vi "InTake Set.vi"(1 "InTake Global Data In":T1) -> (0 "InTake Global Data Out":T1)   [LabVIEW 2013]
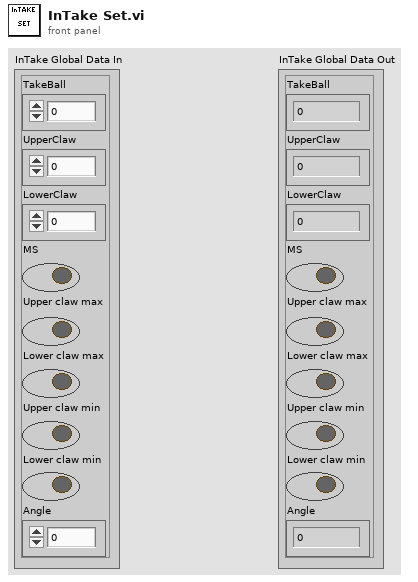
[diagram p1: front panel]
types:
  T1 = cluster{"TakeBall":dbl, "UpperClaw":dbl, "LowerClaw":dbl, "MS":bool, "Upper claw max":bool, "Lower claw max":bool, "Upper claw min":bool, "Lower claw min":bool, "Angle":dbl}
  T2 = typedef "WPI_MotorControlDeviceRef.ctl" = cluster{"DeviceStatus":errorcluster, "Type":enum16{"PWM", "CAN"}, "PWM":cluster{"Digital Module":T3, "PWM Channel":T4, "DeadBand":T5}, "CAN":cluster{"Device Number":u8, "Control Mode":T6, "Semaphore":T7, "Max Vout":dbl}, "Invert":bool, "TransformRef":T8, "InvTransformRef":T8}
  T3 = typedef "FPGA_TypedefDigitalModule.ctl" = enum16{"Digital Module 1", "Digital Module 2"}
  T4 = typedef "FPGA_DIOPWMChannel.ctl" = enum8{"PWM 1", "PWM 2", "PWM 3", "PWM 4", "PWM 5", "PWM 6", "PWM 7", "PWM 8", "PWM 9", "PWM 10", "Invalid"}
  T5 = typedef "WPI_PWMDeadband.ctl" = cluster{"Name":string, "maxPositivePwm":i32, "minPositivePwm":i32, "centerPwm":i32, "maxNegativePwm":i32, "minNegativePwm":i32, "angularRange":u16}
  T6 = typedef "WPI_CANJaguar_ControlMode.ctl" = enum8{"Percent VBus", "Current", "Speed", "Position", "Voltage"}
  T7 = typedef "Semaphore RefNum" = refnum<k1>
  T8 = typedef "WPI_PWMTransform_ConPane.ctl" = refnum<vi>
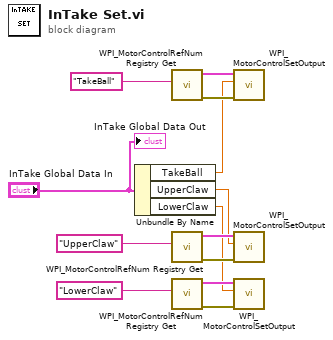
[diagram p0: block diagram]
diagram:
  n1 = Unbundle By Name("InTake Global Data In") -> ("TakeBall"=w10:dbl, "UpperClaw"=w2:dbl, "LowerClaw"=w3:dbl)
  n2 = call <vilib>:"WPI_MotorControlRefNum Registry Get.vi"("refnum name"="TakeBall") -> ("error out"=w12:errorcluster, "MotorControlDevRef"=w13:T2)  [unwired: 9 in]
  n3 = call <vilib>:"WPI_MotorControlRefNum Registry Get.vi"("refnum name"="UpperClaw") -> ("error out"=w9:errorcluster, "MotorControlDevRef"=w8:T2)  [unwired: 9 in]
  n4 = call <vilib>:"WPI_MotorControlRefNum Registry Get.vi"("refnum name"="LowerClaw") -> ("error out"=w4:errorcluster, "MotorControlDevRef"=w5:T2)  [unwired: 9 in]
  n5 = call <vilib>:"WPI_MotorControlSetOutput.vi"("error in (no error)"=w12, "Output"=w10, "MotorControlDevRef"=w13) -> ()  [unwired: 6 in, 3 out]
  n6 = call <vilib>:"WPI_MotorControlSetOutput.vi"("error in (no error)"=w9, "Output"=w2, "MotorControlDevRef"=w8) -> ()  [unwired: 6 in, 3 out]
  n7 = call <vilib>:"WPI_MotorControlSetOutput.vi"("error in (no error)"=w4, "Output"=w3, "MotorControlDevRef"=w5) -> ()  [unwired: 6 in, 3 out]
  "InTake Global Data Out" <- "InTake Global Data In"
